vi "Current Read.vi"   [LabVIEW 2023, in "Device.lvclass"]
uses:
  Device.lvclass
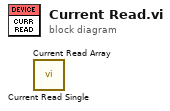
[diagram p0: block diagram]
diagram:
  n1 = call "Current Read Single.vi"() -> ()  [unwired: 9 in, 3 out]
  n2 = call "Current Read Array.vi"() -> ()  [unwired: 10 in, 2 out]
